vi "StudentScope - Voltage Convert.vi"(1 "CH A Scale":u32) -> (0 "Scaled Voltage":dbl)   [LabVIEW 2015]
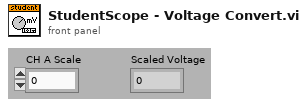
[diagram p1: front panel]
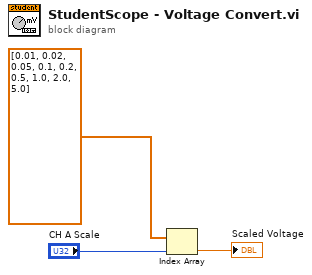
[diagram p0: block diagram]
diagram:
  n1 = Index Array(array=dbl[] [0.01, 0.02, 0.05, 0.1, 0.2, 0.5, 1.0, 2.0, 5.0], index="CH A Scale") -> (element=→"Scaled Voltage":dbl)
